vi "Interlock.vi"() -> (0 "error out":errorcluster)   [LabVIEW 2013]
uses:
  global/InstrumentSetup.vi
panel:
  in  "Error In":errorcluster
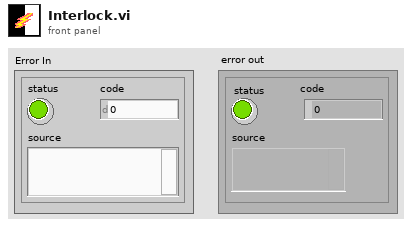
[diagram p1: front panel]
types:
  T1 = cluster{"Edgesense & Temperature":enum16{"Arduino Uno", "Nothing"}, "VISA address":refnum<visa-resource-name>, "VISA address LED array":refnum<visa-resource-name>}
  T2 = cluster{"IV Supply":u16, "GPIB address IV":string, "Bias Supply":u16, "GPIB address Bias":string, "Sensor Bias Voltage [V]":dbl, "IV Supply 2":u16, "GPIB address IV 2":string}
  T3 = cluster{"Volt range":u16, "Compliance":u16, "Readout Flag":u16, "Range:":u16, "Integration:":u16, "Filtering:":u16}
  T4 = cluster{"source/measure (V/I:0)":u16, "function (DC:0)":u16, "DC delay (sec)":dbl, "source range\nI source / V source (auto:0)":u16, "filter (disabled:0)":u16, "integration time (medium:1)":u16, "source level":dbl, "voltage \ncompliance level":dbl, "current \ncompliance level":dbl, "compliance/\nmeasurement range (auto:0)":u16}
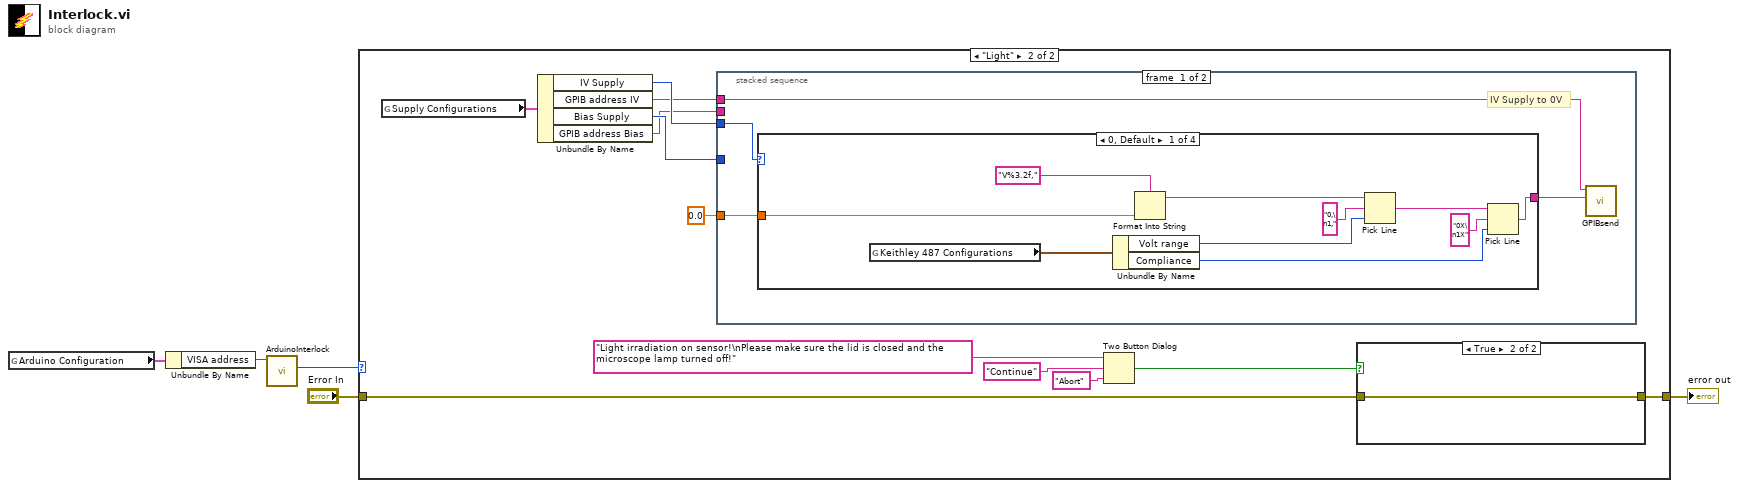
[diagram p0: block diagram]
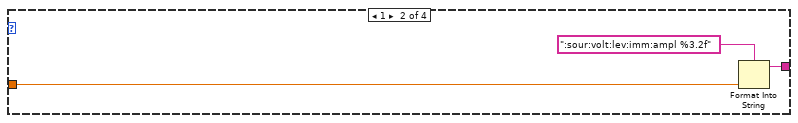
[diagram p3: hidden frame]
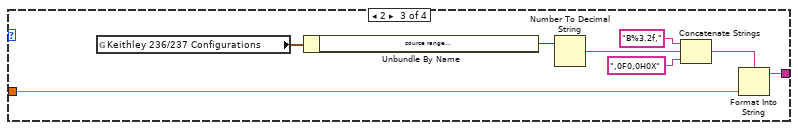
[diagram p4: hidden frame]
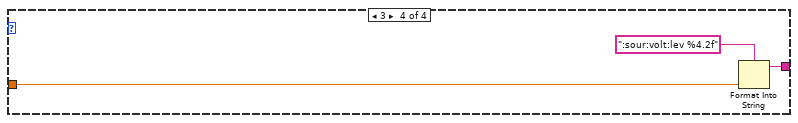
[diagram p5: hidden frame]
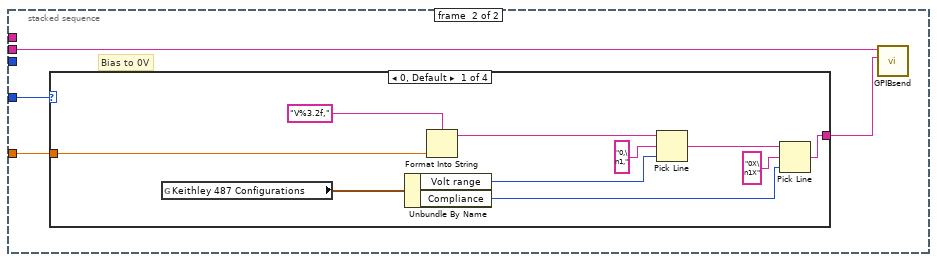
[diagram p6: hidden frame]
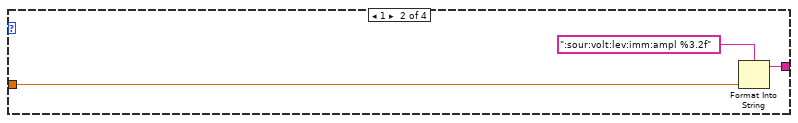
[diagram p7: hidden frame]
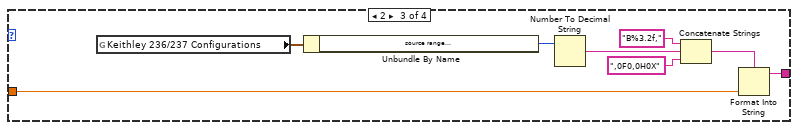
[diagram p8: hidden frame]
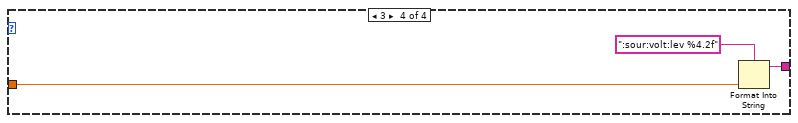
[diagram p9: hidden frame]
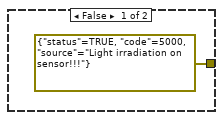
[diagram p10: hidden frame]
diagram:
  n1 = global read "InstrumentSetup.vi" "Arduino Configuration"() -> (w4:T1)
  n2 = Unbundle By Name(w4) -> ("VISA address"=w5:refnum<visa-resource-name>)
  n3 = call "ArduinoInterlock.vi"("VISA resource in"=w5) -> ("Interlock Status"=w3:enum16{"Dark", "Light"})  [unwired: 3 in, 3 out]
  n4 = case shown="\"Light\"" w3 {
    tunnel: "Error In" -> [w6 w7]
    tunnel: [w6 w11] -> w1
    frame "Dark", Default {
    }
    frame "Light" {
      n5 = global read "InstrumentSetup.vi" "Supply Configurations"() -> (w18:T2)
      n6 = Unbundle By Name(w18) -> ("IV Supply"=w17:u16, "GPIB address IV"=w16:string, "Bias Supply"=w15:u16, "GPIB address Bias"=w14:string)
      n7 = stacked-sequence {
        tunnel: 0.0 -> [w19 w47]
        tunnel: w17 -> [w22 _]
        tunnel: w16 -> [w20 _]
        tunnel: w14 -> [_ w49]
        tunnel: w15 -> [_ w48]
        frame #0 {
          # "IV Supply to 0V"
          n8 = case shown="0, Default" w22 {
            tunnel: w19 -> [w32 w35 w43 w46]
            tunnel: [w23 w34 w42 w45] -> w21
            frame 0, Default {
              n9 = global read "InstrumentSetup.vi" "Keithley 487 Configurations"() -> (w31:T3)
              n10 = Unbundle By Name(w31) -> ("Volt range"=w26:u16, "Compliance"=w24:u16)
              n11 = Format Into String(format string="V%3.2f,", w32) -> (resulting string=w25:string)  [unwired: 2 in, 1 out]
              n12 = Pick Line(string ("")=w25, multi-line string="0,\n1,", line index=w26) -> (output string=w28:string)
              n13 = Pick Line(string ("")=w28, multi-line string="0X\n1X", line index=w24) -> (output string=w23:string)
            }
            frame 1 {
              n14 = Format Into String(format string=":sour:volt:lev:imm:ampl %3.2f", w35) -> (resulting string=w34:string)  [unwired: 2 in, 1 out]
            }
            frame 2 {
              n15 = global read "InstrumentSetup.vi" "Keithley 236/237 Configurations"() -> (w41:T4)
              n16 = Unbundle By Name(w41) -> ("source range\nI source / V source (auto:0)"=w40:u16)
              n17 = Number To Decimal String(number=w40) -> (decimal integer string=w37:string)  [unwired: 1 in]
              n18 = Concatenate Strings("B%3.2f,", w37, ",0F0,0H0X") -> (w36:string)
              n19 = Format Into String(format string=w36, w43) -> (resulting string=w42:string)  [unwired: 2 in, 1 out]
            }
            frame 3 {
              n20 = Format Into String(format string=":sour:volt:lev %4.2f", w46) -> (resulting string=w45:string)  [unwired: 2 in, 1 out]
            }
          }
          n21 = call "GPIBsend.vi"("address string"=w20, "write buffer"=w21) -> ()  [unwired: 5 in, 3 out]
        }
        frame #1 {
          # "Bias to 0V"
          n22 = case shown="0, Default" w48 {
            tunnel: [w52 w63 w71 w74] -> w50
            tunnel: w47 -> [w51 w61 w64 w72]
            frame 0, Default {
              n23 = global read "InstrumentSetup.vi" "Keithley 487 Configurations"() -> (w60:T3)
              n24 = Unbundle By Name(w60) -> ("Volt range"=w55:u16, "Compliance"=w53:u16)
              n25 = Format Into String(format string="V%3.2f,", w51) -> (resulting string=w54:string)  [unwired: 2 in, 1 out]
              n26 = Pick Line(string ("")=w54, multi-line string="0,\n1,", line index=w55) -> (output string=w57:string)
              n27 = Pick Line(string ("")=w57, multi-line string="0X\n1X", line index=w53) -> (output string=w52:string)
            }
            frame 1 {
              n28 = Format Into String(format string=":sour:volt:lev:imm:ampl %3.2f", w61) -> (resulting string=w63:string)  [unwired: 2 in, 1 out]
            }
            frame 2 {
              n29 = global read "InstrumentSetup.vi" "Keithley 236/237 Configurations"() -> (w70:T4)
              n30 = Unbundle By Name(w70) -> ("source range\nI source / V source (auto:0)"=w69:u16)
              n31 = Number To Decimal String(number=w69) -> (decimal integer string=w66:string)  [unwired: 1 in]
              n32 = Concatenate Strings("B%3.2f,", w66, ",0F0,0H0X") -> (w65:string)
              n33 = Format Into String(format string=w65, w64) -> (resulting string=w71:string)  [unwired: 2 in, 1 out]
            }
            frame 3 {
              n34 = Format Into String(format string=":sour:volt:lev %4.2f", w72) -> (resulting string=w74:string)  [unwired: 2 in, 1 out]
            }
          }
          n35 = call "GPIBsend.vi"("address string"=w49, "write buffer"=w50) -> ()  [unwired: 5 in, 3 out]
        }
      }
      n36 = Two Button Dialog(message="Light irradiation on sensor!\nPlease make sure the lid is closed and the microscope lamp turned off!", 1:"Abort", 2:"Continue") -> (T button?=w8:bool)
      n37 = case shown="True" w8 {
        tunnel: [errorcluster {"status"=TRUE, "code"=5000, "source"="Light irradiation on sensor!!!"} ("error constant") w76] -> w11
        tunnel: w7 -> [_ w76]
        frame False {
        }
        frame True {
        }
      }
    }
  }
  "error out" <- w1
